vi "Global Chat.vi"(8 "error in (no error)":errorcluster, 10 "Global Msg":string, 11 "Server in":refnum<class "Server.lvclass">) -> (0 "error out":errorcluster, 3 "Server out":refnum<class "Server.lvclass">)   [LabVIEW 2020, in "Server.lvlib" / "Server.lvclass"]
uses:
  Server.lvclass
  Server.lvclass/Server.ctl
  Chat Room Model/Chat Room Model Messages/ReceiveNewMessage Msg/ReceiveNewMessage Msg.lvclass
  Application Control/Message.ctl
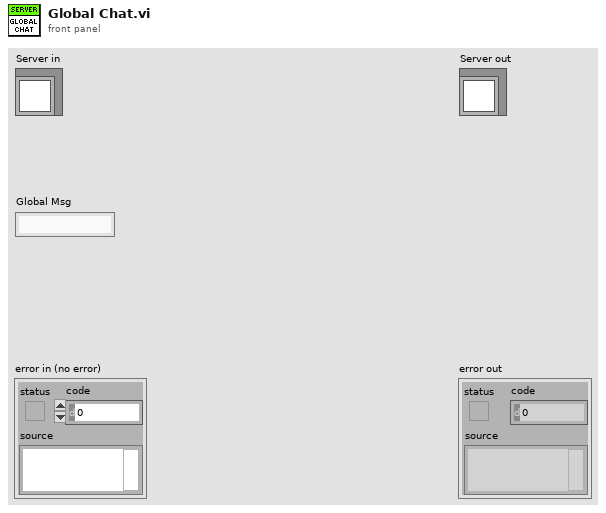
[diagram p1: front panel]
types:
  T1 = typedef "Message.ctl" = cluster{"From":string, "To":string, "Message":string}
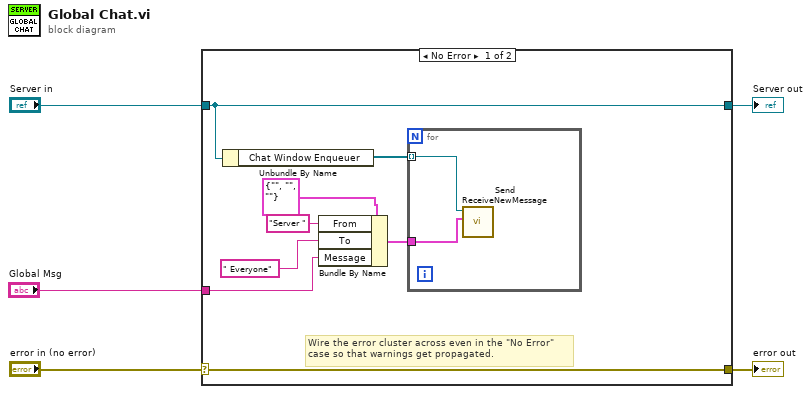
[diagram p0: block diagram]
diagram:
  n1 = case shown="No Error" "error in (no error)" {
    selector: "error in (no error)" -> [w13 w17]
    tunnel: [w13 w17] -> w4
    tunnel: [w12 w16] -> w2
    tunnel: "Server in" -> [w12 w16]
    tunnel: "Global Msg" -> [w8 _]
    frame No Error {
      # "Wire the error cluster across even in the \"No Error\"\ncase so that warnings get propagated."
      n2 = Unbundle By Name(w12) -> ("Chat Window Enqueuer"=w11:refnum<class "Message Enqueuer.lvclass">[])
      n3 = Bundle By Name(cluster=T1 {"From"="", "To"="", "Message"=""} ("Message Cluster"), "From"="Server ", "To"=" Everyone", "Message"=w8) -> (w7:T1)
      n4 = for {
        tunnel: w11 -> [w15] mode=indexing
        tunnel: w7 -> [w14]
        n5 = call "Send ReceiveNewMessage.vi"("Message Cluster"=w14, "Message Enqueuer"=w15) -> ()  [unwired: 8 in, 2 out]
      }
    }
    frame Error {
    }
  }
  "error out" <- w4
  "Server out" <- w2
